vi "loop_timing.vi"(2 "i (reset @ 0)":i32=1) -> (7 "time since start [ms]":i32)   [LabVIEW 2015]
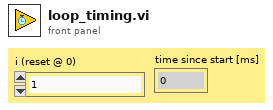
[diagram p1: front panel]
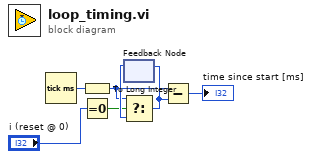
[diagram p0: block diagram]
diagram:
  n1 = Tick Count (ms) ("now")() -> (millisecond timer value=w3:u32)
  n2 = To Long Integer(number=w3) -> (32bit integer=w2:i32)
  n3 = Equal To 0?(x="i (reset @ 0)") -> (x = 0?=w1:bool)
  n4 = feedback #1() -> (w5:i32)  [unwired: 1 in]
  n5 = Select(t=w2, s=w1, f=w5) -> (s? t:f=w4:i32)
  n6 = feedback-in #1(w4) -> ()
  n7 = Subtract(x=w2, y=w4) -> (x-y=→"time since start [ms]":i32)
